vi "Read Waveform Data.vi"(8 "error in (no error)":errorcluster, 11 "Composite Waveform in":refnum<class "Composite Waveform.lvclass">) -> (0 "error out":errorcluster, 2 "Waveform Data":waveform(dbl), 3 "Composite Waveform out":refnum<class "Composite Waveform.lvclass">)   [LabVIEW 2020, in "Composite Waveform.lvclass"]
uses:
  Composite Waveform.lvclass
  Composite Waveform.lvclass/Composite Waveform.ctl
  <vilib>/Waveform/WDTOps.llb/WDT Append Waveforms DBL.vi
  Analog Waveform/Analog Waveform.lvclass
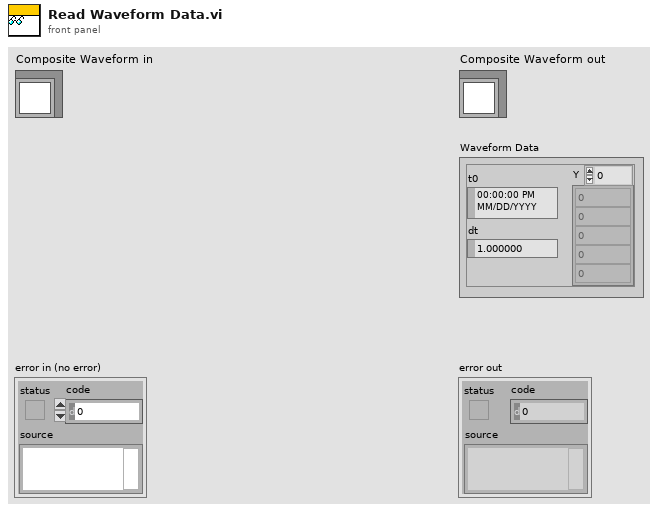
[diagram p1: front panel]
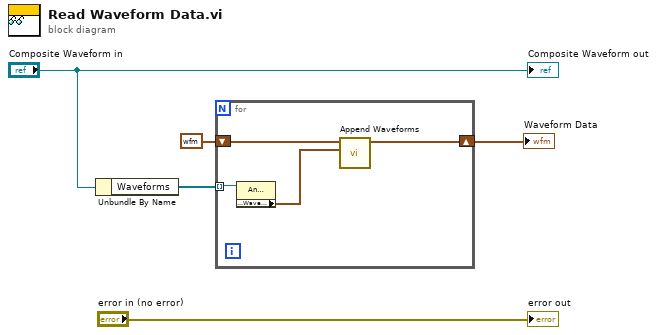
[diagram p0: block diagram]
diagram:
  n1 = Unbundle By Name("Composite Waveform in") -> ("Waveforms"=w3:refnum<class "Analog Waveform.lvclass">[])
  n2 = for {
    tunnel: w3 -> [w9] mode=indexing
    shift-right: [w7] -> w1
    shift-left: waveform(dbl) {"t0"=timestamp(0 s since 1904-01-01), "dt"=1.0, "Y"=[]} ("Waveform") -> [w6]
    n3 = property class="Analog Waveform.lvclass"(reference=w9) -> ("Member Accessors:Waveform Data"=w8:waveform(dbl))  [unwired: 1 in, 2 out]
    n4 = call-poly <vilib>:"Append Waveforms.vi"("waveform B"=w8, "waveform A"=w6) -> ("waveform out"=w7:waveform(dbl))  [unwired: 8 in, 1 out]
  }
  "Waveform Data" <- w1
  "error out" <- "error in (no error)"
  "Composite Waveform out" <- "Composite Waveform in"
